vi "Restart Camera server.vi"() -> (0 "Error Out":errorcluster)   [LabVIEW 2015]
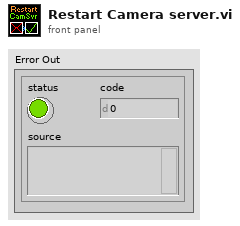
[diagram p1: front panel]
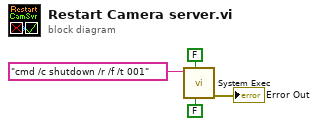
[diagram p0: block diagram]
diagram:
  n1 = call <vilib>:"System Exec.vi"("run minimized? (F)"=FALSE, "wait until completion? (T)"=FALSE, "command line"="cmd /c shutdown /r /f /t 001") -> ("error out"=→"Error Out":errorcluster)  [unwired: 5 in, 3 out]
